vi "convert old sequence step def to latest_string.vi"(8 "error in":errorcluster, 11 "data string":string) -> (0 "error out":errorcluster, 3 "RSLinx String Cluster out":T1={"Data String"="", "PLC Path and Tag"={"Tag Name"="", "Network Path"="", "use opc"=FALSE, "DataSocket Reference"={"CWDSLib._DCWDataSocket"=refnum, "CWDSLib._DCWData"=refnum, "OnDataUpdated"=0, "OnStatusUpdated"=0}}, "Error No."=157, "timeout (ms)"=10000} {"PLC Path and Tag"."DataSocket Reference"."OnStatusUpdated" format="%.0x"; "PLC Path and Tag"."DataSocket Reference"."OnDataUpdated" format="%.0x"})   [LabVIEW 2018]
uses:
  type defs/RSLinx String Cluster.ctl
  type defs/plc path and tag.ctl
  <vilib>/Platform/dataskt.llb/DataSocket Reference Type.ctl
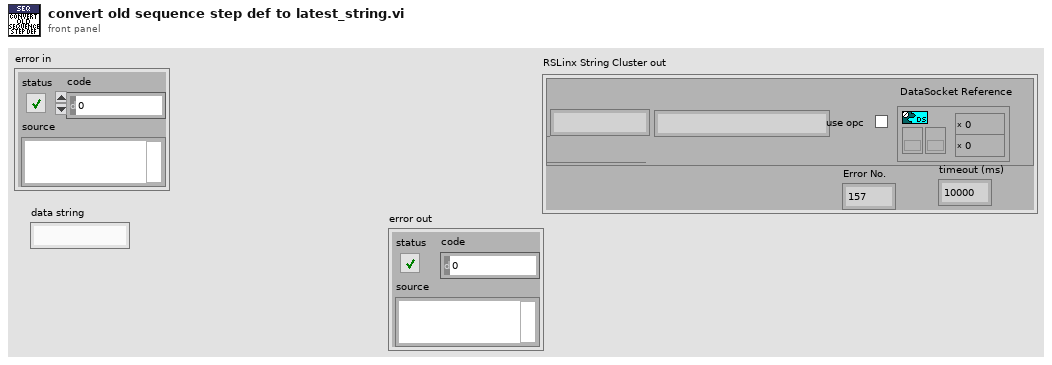
[diagram p1: front panel]
types:
  T1 = typedef "RSLinx String Cluster.ctl" = cluster{"Data String":string, "PLC Path and Tag":T2, "Error No.":u16, "timeout (ms)":i32}
  T2 = typedef "plc path and tag.ctl" = cluster{"Tag Name":string, "Network Path":string, "use opc":bool, "DataSocket Reference":T3}
  T3 = typedef "DataSocket Reference Type.ctl" = cluster{"CWDSLib._DCWDataSocket":refnum<k7>, "CWDSLib._DCWData":refnum<k7>, "OnDataUpdated":u32, "OnStatusUpdated":u32}
  T4 = cluster{"Data String":string, "PLC Path and Tag":cluster{"Tag Name":string, "Network Path":string, "use opc":bool, "DataSocket Reference":cluster{"CWDSLib._DCWDataSocket":refnum<k7>, "CWDSLib._DCWData":refnum<k7>, "OnDataUpdated":u32, "OnStatusUpdated":u32}}, "Error No.":u16}
  T5 = cluster{"Tag Name":string, "Network Path":string, "use opc":bool, "DataSocket Reference":cluster{"CWDSLib._DCWDataSocket":refnum<k7>, "CWDSLib._DCWData":refnum<k7>, "OnDataUpdated":u32, "OnStatusUpdated":u32}}
  T6 = cluster{"Data String":string, "PLC Path and Tag":T2}
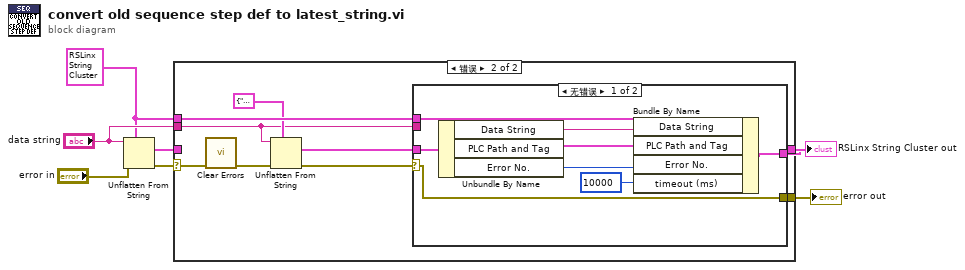
[diagram p0: block diagram]
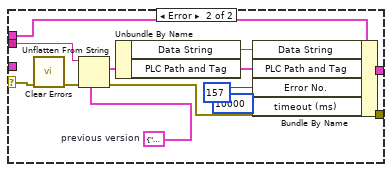
[diagram p3: hidden frame]
diagram:
  w3 = T1 {"Data String"="", "PLC Path and Tag"={"Tag Name"="", "Network Path"="", "use opc"=FALSE, "DataSocket Reference"={"CWDSLib._DCWDataSocket"=refnum, "CWDSLib._DCWData"=refnum, "OnDataUpdated"=0, "OnStatusUpdated"=0}}, "Error No."=157, "timeout (ms)"=0} ("RSLinx String Cluster in")
  n1 = Unflatten From String(type=w3, binary string="data string", error in (no error)="error in") -> (value=w5:T1, error out=w7:errorcluster)  [unwired: 2 in, 1 out]
  n2 = case shown="错误" w7 {
    selector: w7 -> [w8 w14]
    tunnel: [w9 w17] -> w6
    tunnel: w5 -> [w9 _]
    tunnel: "data string" -> [_ w12]
    tunnel: w3 -> [_ w18]
    tunnel: [w8 w16] -> w1
    frame No Error {
    }
    frame Error {
      n3 = call <vilib>:"Clear Errors.vi"("error in (no error)"=w14) -> ("error out"=w15:errorcluster)  [unwired: 5 in, 1 out]
      n4 = Unflatten From String(type=T4 {"Data String"="", "PLC Path and Tag"={"Tag Name"="", "Network Path"="", "use opc"=FALSE, "DataSocket Reference"={"CWDSLib._DCWDataSocket"=refnum, "CWDSLib._DCWData"=refnum, "OnDataUpdated"=0, "OnStatusUpdated"=0}}, "Error No."=157} ("RSLinx String Cluster in"), binary string=w12, error in (no error)=w15) -> (value=w10:T4, error out=w11:errorcluster)  [unwired: 2 in, 1 out]
      n5 = case shown="无错误" w11 {
        selector: w11 -> [w23 w28]
        tunnel: w18 -> [w25 w37]
        tunnel: [w24 w36] -> w17
        tunnel: [w23 w31] -> w16
        tunnel: w12 -> [_ w29]
        tunnel: w10 -> [w26 _]
        frame No Error {
          n6 = Unbundle By Name(w26) -> ("Data String"=w22:string, "PLC Path and Tag"=w21:T5, "Error No."=w20:u16)
          n7 = Bundle By Name(cluster=w25, "Data String"=w22, "PLC Path and Tag"=w21, "Error No."=w20, "timeout (ms)"=10000) -> (w24:T1)
        }
        frame Error {
          w38 = T6 {"Data String"="", "PLC Path and Tag"={"Tag Name"="", "Network Path"="", "use opc"=FALSE, "DataSocket Reference"={"CWDSLib._DCWDataSocket"=refnum, "CWDSLib._DCWData"=refnum, "OnDataUpdated"=0, "OnStatusUpdated"=0}}}  # previous version
          n8 = call <vilib>:"Clear Errors.vi"("error in (no error)"=w28) -> ("error out"=w30:errorcluster)  [unwired: 5 in, 1 out]
          n9 = Unflatten From String(type=w38, binary string=w29, error in (no error)=w30) -> (value=w35:T6, error out=w31:errorcluster)  [unwired: 2 in, 1 out]
          n10 = Unbundle By Name(w35) -> ("Data String"=w34:string, "PLC Path and Tag"=w33:T2)
          n11 = Bundle By Name(cluster=w37, "Data String"=w34, "PLC Path and Tag"=w33, "Error No."=u16 157, "timeout (ms)"=10000) -> (w36:T1)
        }
      }
    }
  }
  "RSLinx String Cluster out" <- w6
  "error out" <- w1
